vi "ui_DataLog Reorder Listed Strings.vi"(0 "prompt":string, 7 "list of strings":string[](array[string])) -> (4 "OKed?":bool, 8 "reordered strings":string[](array[string]))   [LabVIEW 2012]
doc: "Allows a set of strings to be reordered. The strings are displayed in a list whose items can be dragged so as to change their order."
uses:
  typedefs/t_DataLog Reorder Listed Strings States.ctl
panel:
  in  "list":i32(listbox) caption="drag items into the desired order"
  in  "cancel":bool
  in  "OK":bool
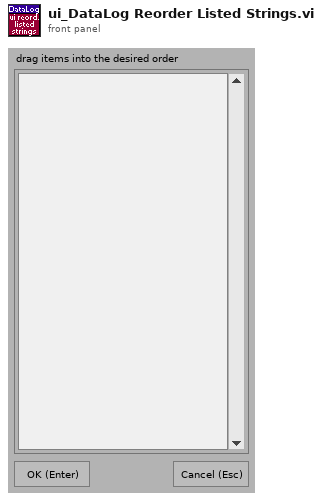
[diagram p1: front panel]
types:
  T1 = typedef "t_DataLog Reorder Listed Strings States.ctl" = enum16{"empty queue", "initialize", "init controls", "init check list", "init list", "cleanup", "stop"}
  T2 = typedef "eventvkey.ctl" = enum16{"ASCII", "Enter", "Return", "Shift", "Ctrl", "Alt", "Cmd", "Opt", "Caps", "NumLock", "Clear", "Break", "Up", "Down", "Left", "Right", "Insert", "Delete", "Home", "End", "PageUp", "PageDown", "Escape", "Help", "Pause", "ScrollLock", "F1", "F2", "F3", "F4", "F5", "F6", "F7", "F8", "F9", "F10", "F11", "F12", "F13", "F14", "F15", "F16", "F17", "F18", "F19", "F20", "F21", "F22", "F23", "F24", "Play", "VolumeUp", "VolumeDown", "Mute", "Two Byte Char"}
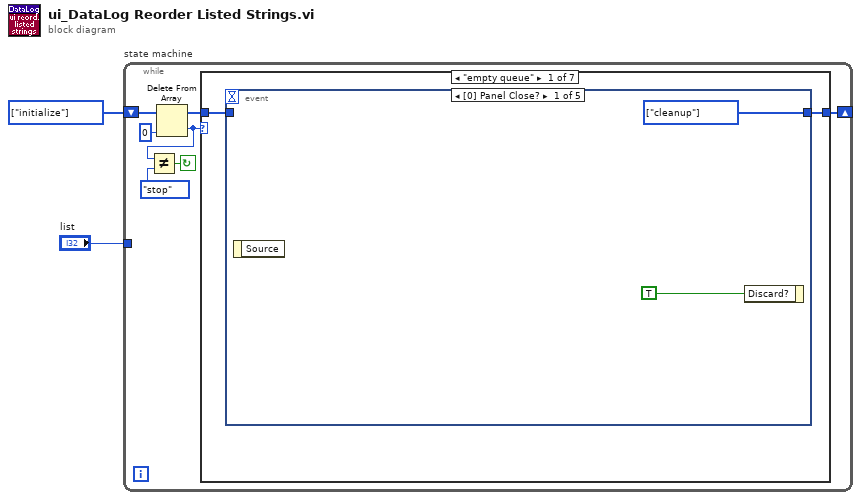
[diagram p0: block diagram]
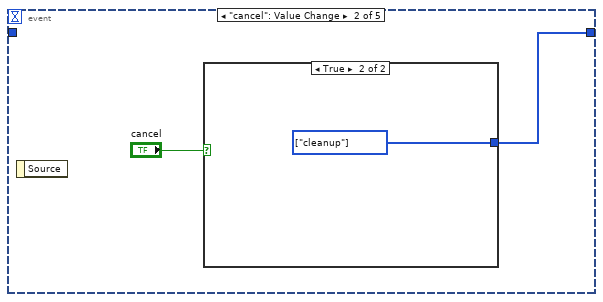
[diagram p2: hidden frame]
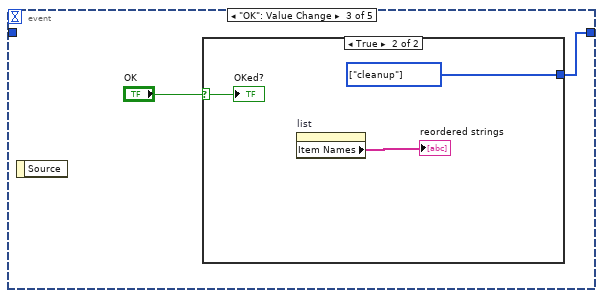
[diagram p4: hidden frame]
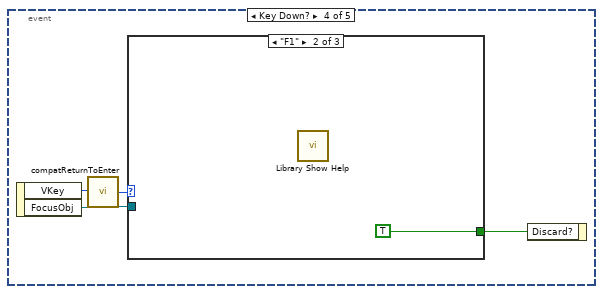
[diagram p6: hidden frame]
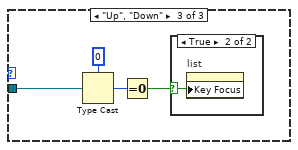
[diagram p8: hidden frame]
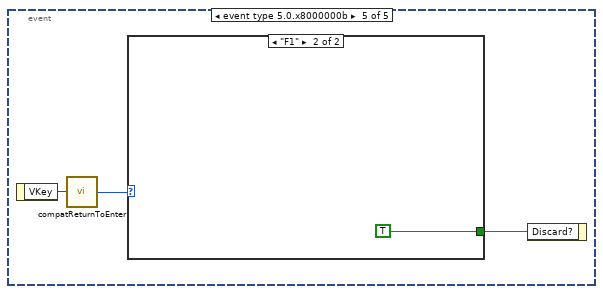
[diagram p10: hidden frame]
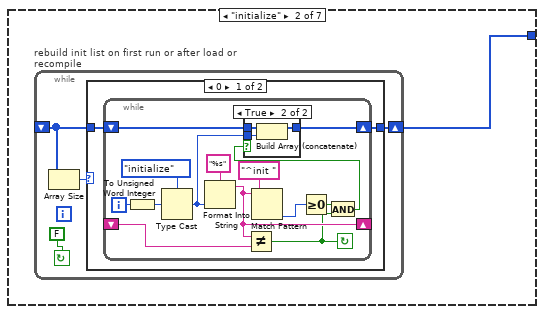
[diagram p12: hidden frame]
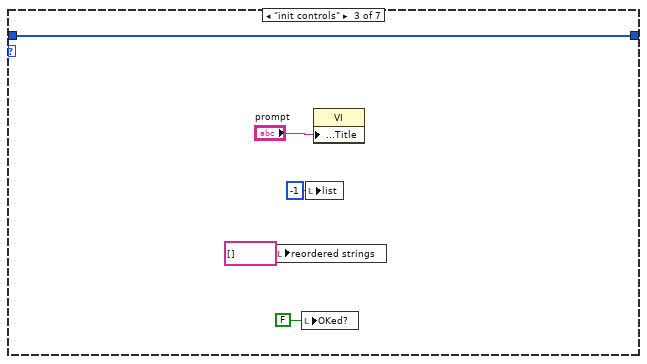
[diagram p15: hidden frame]
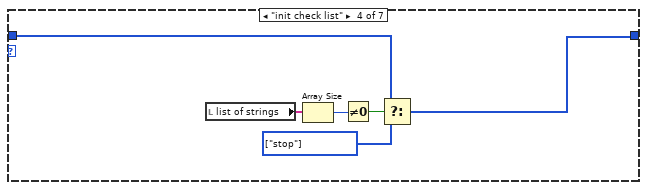
[diagram p16: hidden frame]
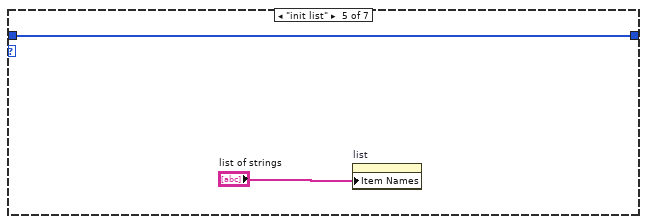
[diagram p17: hidden frame]
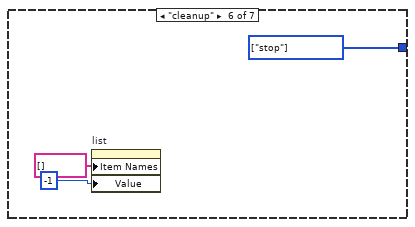
[diagram p18: hidden frame]
diagram:
  w2 = T1[] [enum."initialize"] items=["empty queue", "initialize", "init controls", "init check list", "init list", "cleanup", "stop"] ("Array Constant")
  n1 = while "state machine" {
    shift-left: w2 -> [w6]
    shift-right: [w9] -> _
    tunnel: "list" -> [_]
    stop <- w8 continue-if-true
    n2 = Delete From Array(array=w6, index=0) -> (deleted portion=w3:T1, array with subset deleted=w5:T1[])  [unwired: 1 in]
    n3 = Not Equal?(x=w3, y=t_DataLog_Reorder_Listed_Strings_States."stop" ("states")) -> (x != y?=w8:bool)
    n4 = case "Case" shown="\"empty queue\"" w3 {
      tunnel: [w11 w36 w66 w68 w74 w77 w78] -> w9
      tunnel: w5 -> [w10 _ w66 w69 w74 _ w78]
      frame "empty queue" {
        n5 = event shown="[0] Panel Close?" {
          selector: _ -> [_ _ _ _ _]
          dyn-events: _ -> [_ _ _ _ _]
          timeout: _ -> [_ _ _ _ _]
          tunnel: [w13 w14 w18 _ _] -> w11
          tunnel: w10 -> [_ _ _ _ _]
          event Panel Close? {
            w13 = T1[] [enum."cleanup"] items=["empty queue", "initialize", "init controls", "init check list", "init list", "cleanup", "stop"] ("Array Constant")
            n6 = event-data() -> ()  [unwired: 1 in, 1 out]
            n7 = event-data("Discard?"=TRUE) -> ()  [unwired: 1 in, 1 out]
          }
          event "cancel": Value Change {
            n8 = event-data() -> ()  [unwired: 1 in, 1 out]
            n9 = case shown="True" "cancel" {
              tunnel: [_ w16] -> w14
              frame False {
              }
              frame True {
                w16 = T1[] [enum."cleanup"] items=["empty queue", "initialize", "init controls", "init check list", "init list", "cleanup", "stop"] ("Array Constant")
              }
            }
          }
          event "OK": Value Change {
            n10 = event-data() -> ()  [unwired: 1 in, 1 out]
            n11 = case shown="True" "OK" {
              selector: "OK" -> [_ w20]
              tunnel: [_ w21] -> w18
              frame False {
              }
              frame True {
                w21 = T1[] [enum."cleanup"] items=["empty queue", "initialize", "init controls", "init check list", "init list", "cleanup", "stop"] ("Array Constant")
                n12 = property on="list" class="LstBox (strict)"() -> ("Item Names"=→"reordered strings":string[])  [unwired: 2 in, 2 out]
                "OKed?" <- w20
              }
            }
          }
          event Key Down? {
            n13 = event-data() -> ("VKey"=w22:T2, "FocusObj"=w23:refnum<vi>)  [unwired: 1 in]
            n14 = call <vilib>:"compatReturnToEnter.vi"("VKey"=w22) -> ("VKey"=w25:T2)
            n15 = case shown="\"F1\"" w25 {
              tunnel: [_ TRUE ("Discard?") _] -> w24
              tunnel: w23 -> [_ _ w28]
              frame Default {
              }
              frame "F1" {
                n16 = call "Library Show Help.vi"() -> ()  [unwired: 1 in]
              }
              frame "Up", "Down" {
                n17 = Type Cast(type=0, x=w28) -> (*(type *) &x=w30:i32)
                n18 = Equal To 0?(x=w30) -> (x = 0?=w27:bool)
                n19 = case shown="True" w27 {
                  selector: w27 -> [_ w31]
                  frame False {
                  }
                  frame True {
                    n20 = property on="list" class="LstBox (strict)"("Key Focus"=w31) -> ()  [unwired: 2 in, 2 out]
                  }
                }
              }
            }
            n21 = event-data("Discard?"=w24) -> ()  [unwired: 1 in, 1 out]
          }
          event event type 5.0.x8000000b {
            n22 = event-data() -> ("VKey"=w32:T2)  [unwired: 1 in]
            n23 = call <vilib>:"compatReturnToEnter.vi"("VKey"=w32) -> ("VKey"=w34:T2)
            n24 = case shown="\"F1\"" w34 {
              tunnel: [_ TRUE ("Discard?")] -> w33
              frame Default {
              }
              frame "F1" {
              }
            }
            n25 = event-data("Discard?"=w33) -> ()  [unwired: 1 in, 1 out]
          }
        }
      }
      frame "initialize" {
        n26 = while "rebuild init list on first run or after load or recompile" {
          shift-left: _ -> [w39]
          shift-right: [w38] -> w36
          stop <- FALSE continue-if-true
          n27 = Array Size(array=w39) -> (size(s)=w40:i32)
          n28 = case shown="0" w40 {
            tunnel: [w41 w61] -> w38
            tunnel: w39 -> [w42 w61]
            frame 0 {
              n29 = while {
                shift-left: w42 -> [w51]
                shift-right: [w49] -> w41
                shift-left: _ -> [w53]
                shift-right: [w48] -> _
                i -> [w56]
                stop <- w44 continue-if-true
                n30 = To Unsigned Word Integer(number=w56) -> (unsigned 16bit integer=w54:u16)
                n31 = Type Cast(type=t_DataLog_Reorder_Listed_Strings_States."initialize" ("states"), x=w54) -> (*(type *) &x=w50:T1)
                n32 = Format Into String(format string="%s" ("Format String"), w50) -> (resulting string=w48:string)  [unwired: 2 in, 1 out]
                n33 = Not Equal?(x=w48, y=w53) -> (x != y?=w44:bool)
                n34 = Match Pattern(string=w48, regular expression="^init ") -> (offset past match=w46:i32)  [unwired: 1 in, 3 out]
                n35 = Greater Or Equal To 0?(x=w46) -> (x >= 0?=w45:bool)
                n36 = And(x=w45, y=w44) -> (x .and. y?=w43:bool)
                n37 = case shown="True" w43 {
                  tunnel: w51 -> [w57 w60]
                  tunnel: w50 -> [_ w59]
                  tunnel: [w57 w58] -> w49
                  frame False {
                  }
                  frame True {
                    n38 = Build Array (concatenate)(w60, w59) -> (w58:T1[])
                  }
                }
              }
            }
            frame Default {
            }
          }
        }
      }
      frame "init controls" {
        n39 = local write "reordered strings"(string[] [] ("reodered strings")) -> ()
        n40 = local write "OKed?"(FALSE ("OKed?")) -> ()
        n41 = local write "list"(-1 ("list")) -> ()
        n42 = property class="VI"("Front Panel Window:Title"="prompt") -> ()  [unwired: 2 in, 2 out]
      }
      frame "init check list" {
        w70 = T1[] [enum."stop"] items=["empty queue", "initialize", "init controls", "init check list", "init list", "cleanup", "stop"] ("Array Constant")
        n43 = local read "list of strings"() -> (w67:string[])
        n44 = Array Size(array=w67) -> (size(s)=w72:i32)
        n45 = Not Equal To 0?(x=w72) -> (x != 0?=w71:bool)
        n46 = Select(t=w69, s=w71, f=w70) -> (s? t:f=w68:T1[])
      }
      frame "init list" {
        n47 = property on="list" class="LstBox (strict)"("Item Names"="list of strings") -> ()  [unwired: 2 in, 2 out]
      }
      frame "cleanup" {
        w77 = T1[] [enum."stop"] items=["empty queue", "initialize", "init controls", "init check list", "init list", "cleanup", "stop"] ("Array Constant")
        n48 = property on="list" class="LstBox (strict)"("Item Names"=string[] [], "Value"=-1 ("list")) -> ()  [unwired: 2 in, 2 out]
      }
      frame "stop" {
      }
    }
  }
